vi "Init.vi"(8 "error in (no error)":errorcluster, 11 "AverageCollector2D in":refnum<class "AverageCollector2D.lvclass">) -> (0 "error out":errorcluster, 3 "AverageCollector2D out":refnum<class "AverageCollector2D.lvclass">)   [LabVIEW 2014, in "AverageCollector2D.lvclass"]
uses:
  AverageCollector2D.lvclass
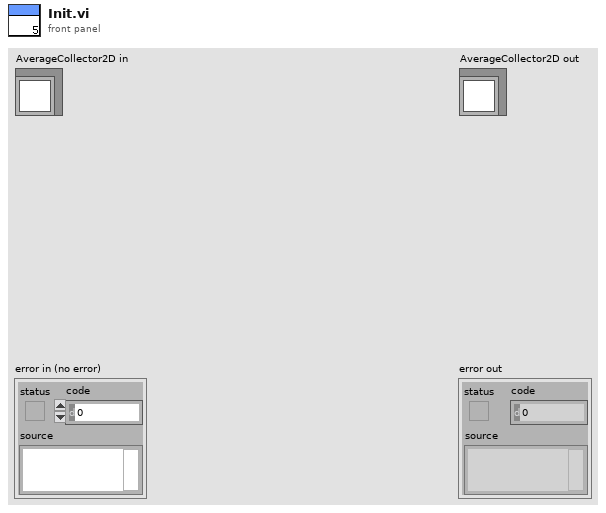
[diagram p1: front panel]
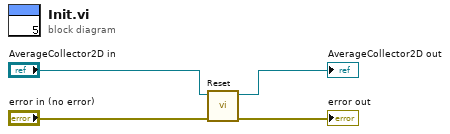
[diagram p0: block diagram]
diagram:
  n1 = call-dynamic "Reset.vi"("error in (no error)"="error in (no error)", "AbstractCollector2D in"="AverageCollector2D in") -> ("error out"=→"error out":errorcluster, "AbstractCollector2D out"=→"AverageCollector2D out":refnum<class "AverageCollector2D.lvclass">)  [unwired: 8 in]
